vi "Search for Virtual Folder.vi"(10 "Virtual Folder":string, 11 "Project Refnum":refnum<vi>) -> (0 "Best Match Name":string, 1 "matched?":bool, 2 "best match":refnum<vi>, 3 "All matches":refnum<vi>[](array[refnum]))   [LabVIEW 2013, in "Caraya.lvlib" / "Test Runner.Project.lvclass"]
uses:
  Test Runner.Project.lvclass
panel:
  out "search string":string
  out "All folders":string[](array[string])
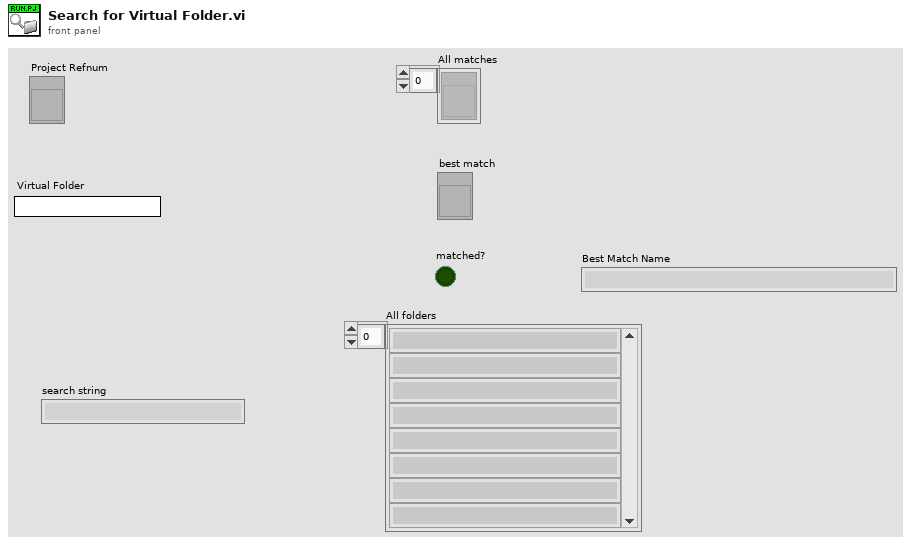
[diagram p1: front panel]
types:
  T1 = cluster{"Project Item":refnum<vi>, "Path":string[]}
  T2 = cluster{"Project Item":refnum<vi>, "Path":string[]}[]
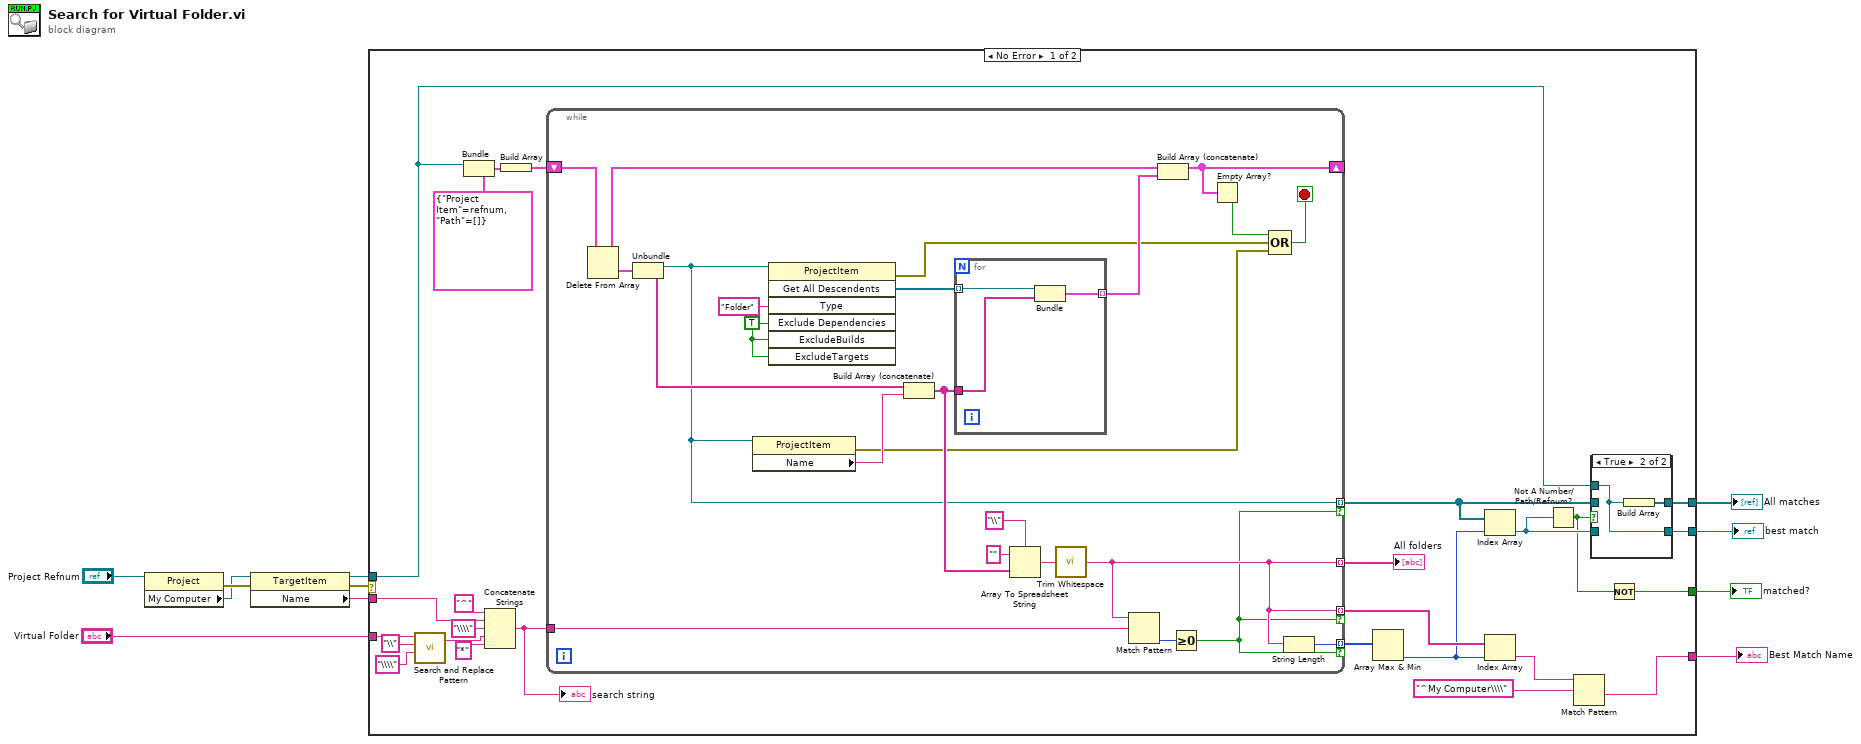
[diagram p0: block diagram]
diagram:
  n1 = property on="Property Node" class="Project"(reference="Project Refnum") -> (error out=w5:errorcluster, "My Computer"=w4:refnum<vi>)  [unwired: 1 in, 1 out]
  n2 = property on="Property Node" class="TargetItem"(reference=w4, error in=w5) -> (reference out=w3:refnum<vi>, error out=w2:errorcluster, "Name"=w8:string)
  n3 = case shown="No Error" w2 {
    tunnel: "Virtual Folder" -> [w18 _]
    tunnel: [w12 _] -> w10
    tunnel: w8 -> [w26 _]
    tunnel: [w25 w69] -> w7
    tunnel: [w23 _] -> w6
    tunnel: w3 -> [w21 w69]
    tunnel: [w15 _] -> w1
    frame No Error {
      n4 = call <vilib>:"Search and Replace Pattern.vi"("string"=w18, "regular expression (\"\")"="\\" ("string"), "replace string (\"\")"="\\\\" ("string")) -> ("result string"=w17:string)  [unwired: 2 in, 1 out]
      n5 = Bundle(cluster=T1 {"Project Item"=refnum, "Path"=[]}, "Project Item"=w21) -> (w36:T1)  [unwired: 1 in]
      n6 = Concatenate Strings("^" ("string"), w26, "\\\\" ("string"), w17, "*" ("string")) -> (w33:string)
      "search string" <- w33
      n7 = Build Array(w36) -> (w37:T2)
      n8 = while {
        shift-right: [w58] -> _
        shift-left: w37 -> [w65]
        tunnel: [w46] -> w22 mode=indexing if=w47
        tunnel: [w49] -> w34 mode=indexing
        tunnel: w33 -> [w51]
        tunnel: [w49] -> w29 mode=indexing if=w47
        tunnel: [w48] -> w30 mode=indexing if=w47
        stop <- w44 stop-if-true
        w63 = TRUE ("ExcludeDependencies")
        n9 = Delete From Array(array=w65) -> (deleted portion=w62:T1, array with subset deleted=w59:T2)  [unwired: 2 in]
        n10 = Unbundle(w62) -> ("Project Item"=w46:refnum<vi>, "Path"=w61:string[])
        n11 = property on="Property Node" class="ProjectItem"(reference=w46) -> (error out=w43:errorcluster, "Name"=w60:string)  [unwired: 1 in, 1 out]
        n12 = invoke class="ProjectItem" method="Get All Descendents"(reference=w46, "Type"="Folder", "Exclude Dependencies"=w63, "ExcludeBuilds"=w63, "ExcludeTargets"=w63) -> (error out=w42:errorcluster, "All Descendents"=w57:refnum<vi>[])  [unwired: 2 in, 5 out]
        n13 = Build Array (concatenate)(w61, w60) -> (w55:string[])
        n14 = for {
          tunnel: w57 -> [w68] mode=indexing
          tunnel: [w67] -> w56 mode=indexing
          tunnel: w55 -> [w66]
          n15 = Bundle(w68, w66) -> (w67:cluster{refnum<vi>, string[]})  [unwired: 1 in]
        }
        n16 = Array To Spreadsheet String(delimiter (Tab)="\\", array=w55, 3:"" ("format string")) -> (spreadsheet string=w52:string)
        n17 = call <vilib>:"Trim Whitespace.vi"("string"=w52) -> ("trimmed string"=w49:string)  [unwired: 1 in]
        n18 = Match Pattern(string=w49, regular expression=w51) -> (offset past match=w50:i32)  [unwired: 1 in, 3 out]
        n19 = Build Array (concatenate)(w59, w56) -> (w58:T2)
        n20 = Greater Or Equal To 0?(x=w50) -> (x >= 0?=w47:bool)
        n21 = Empty Array?(array=w58) -> (empty?=w45:bool)
        n22 = Compound Arithmetic op=OR(w45, w42, w43) -> (w44:bool)
        n23 = String Length(string=w49) -> (length=w48:i32)
      }
      "All folders" <- w34
      n24 = Array Max & Min(array=w30) -> (min index (indices)=w28:i32)  [unwired: 3 out]
      n25 = Index Array(array=w22, index=w28) -> (element=w24:refnum<vi>)
      n26 = Index Array(array=w29, index=w28) -> (element=w13:string)
      n27 = Not A Number/Path/Refnum?(number/path/refnum=w24) -> (NaN/Path/Refnum?=w16:bool)
      n28 = Match Pattern(string=w13, regular expression="^My Computer\\\\" ("string")) -> (after substring=w12:string)  [unwired: 1 in, 3 out]
      n29 = case shown="True" w16 {
        tunnel: w21 -> [_ w40]
        tunnel: [w39 w40] -> w25
        tunnel: w24 -> [w39 _]
        tunnel: [w38 w41] -> w23
        tunnel: w22 -> [w38 _]
        frame False {
        }
        frame True {
          n30 = Build Array(w40) -> (w41:refnum<vi>[])
        }
      }
      n31 = Not(x=w16) -> (.not. x?=w15:bool)
    }
    frame Error {
    }
  }
  "Best Match Name" <- w10
  "All matches" <- w6
  "best match" <- w7
  "matched?" <- w1
